vi "参考-分析生成报告文件.vi"(1 "最大缺陷面积":dbl, 2 "分析结果字符串":string[][](table), 3 "总缺陷面积":dbl, 4 "检测面  是否合格":string, 5 "请输入当前工件型号":string, 6 "时间":string) -> (0 "输出":string)   [LabVIEW 2018]
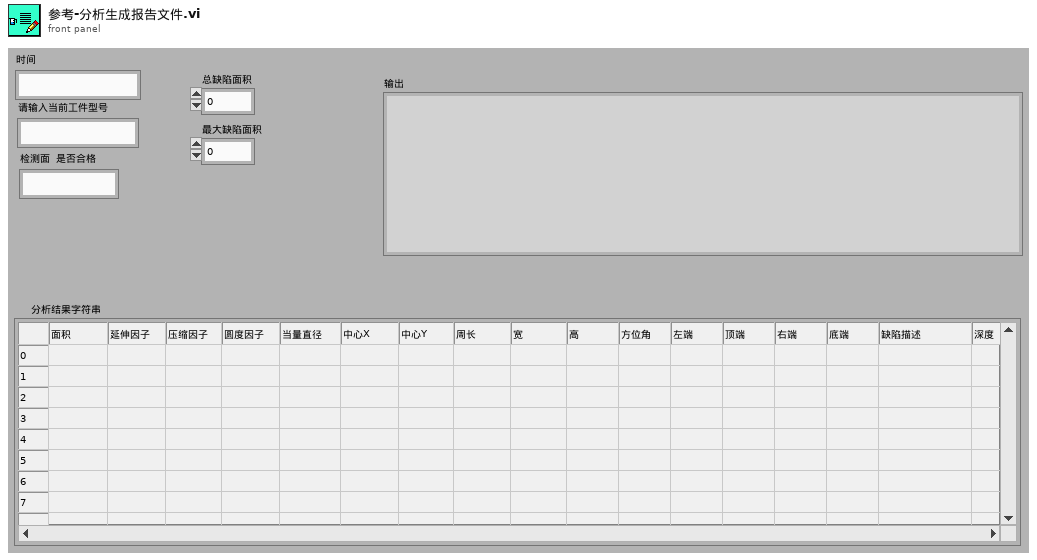
[diagram p1: front panel]
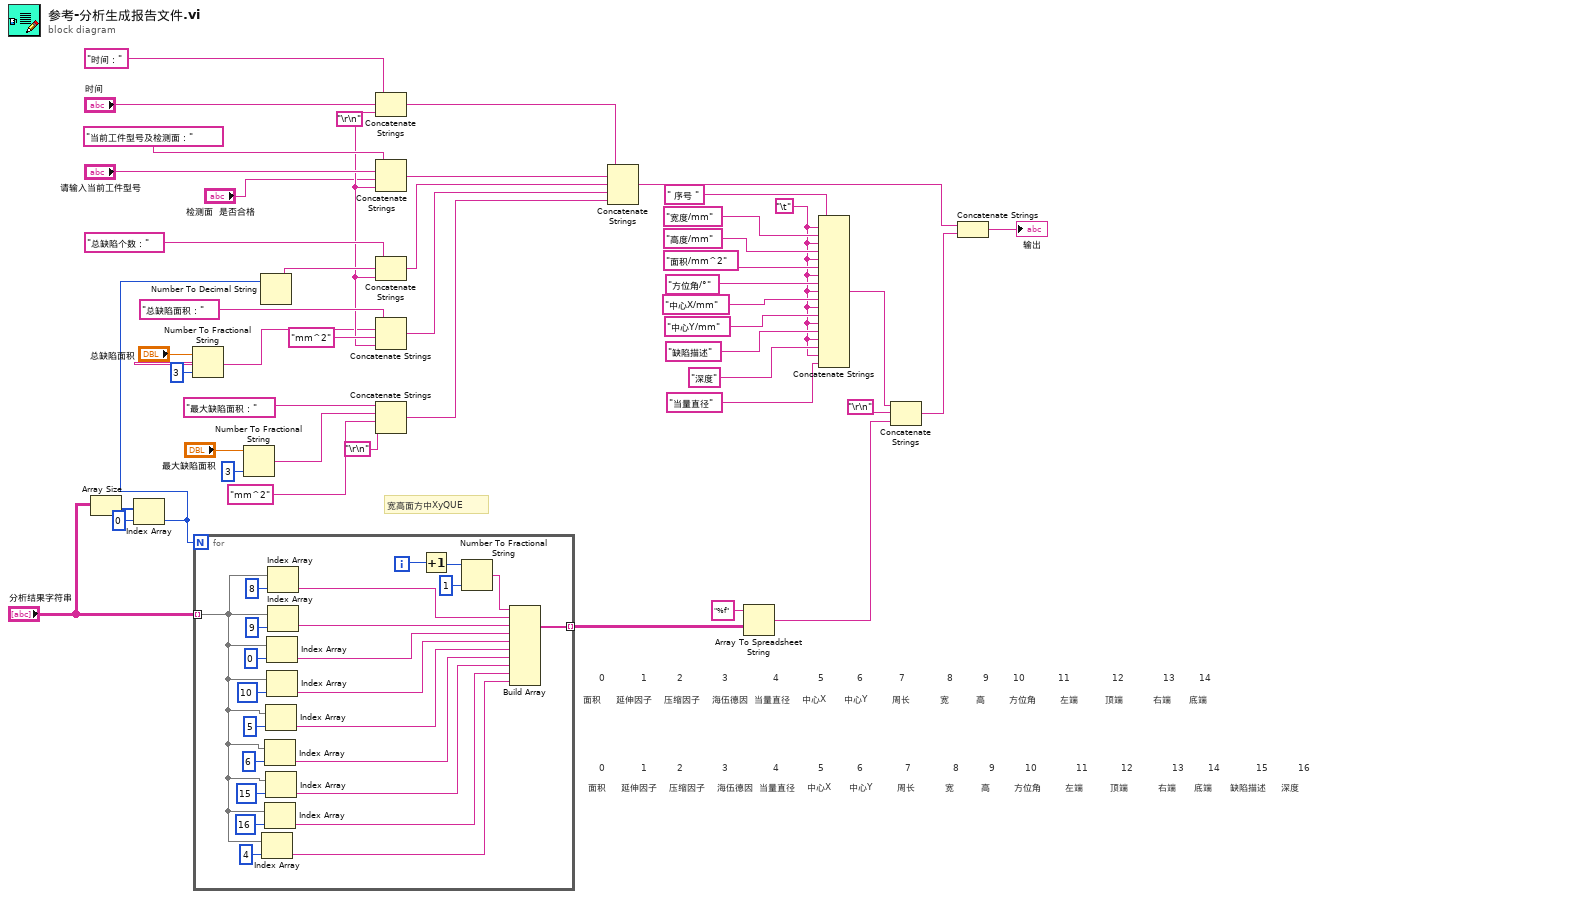
[diagram p0: block diagram]
diagram:
  w2 = "\t"
  w23 = "\r\n"
  # "面积     延伸因子    压缩因子    海伍德因  当量直径    中心X      中心Y        周长          宽         高        方位角        左端         顶端          右端      底端      缺陷描述     深度"
  # "0            1          2             3               4             5           6              7              8          9          10             11           12             13        14            15          16"
  # "面积     延伸因子    压缩因子    海伍德因  当量直径    中心X      中心Y        周长          宽         高        方位角        左端         顶端          右端      底端"
  # "0            1          2             3               4             5           6            7              8          9        10           11              12             13        14"
  # "宽高面方中XyQUE"
  n1 = Array Size(array="分析结果字符串") -> (size(s)=w6:i32[])
  n2 = Index Array(array=w6, index=0 ("索引")) -> (element=w4:i32)
  n3 = Number To Fractional String(number="总缺陷面积", precision (6)=i16 3) -> (F-format string=w20:string)  [unwired: 2 in]
  n4 = for {
    N: w4 -> [_]
    tunnel: [w71] -> w8 mode=indexing
    tunnel: "分析结果字符串" -> [w50] mode=indexing
    i -> [w70]
    n5 = Index Array(array=w50, index=4 ("索引")) -> (element=w49:string)
    n6 = Index Array(array=w50, index=6 ("索引")) -> (element=w55:string)
    n7 = Index Array(array=w50, index=16 ("索引")) -> (element=w48:string)
    n8 = Index Array(array=w50, index=5 ("索引")) -> (element=w56:string)
    n9 = Index Array(array=w50, index=15 ("索引")) -> (element=w53:string)
    n10 = Index Array(array=w50, index=0 ("索引")) -> (element=w61:string)
    n11 = Index Array(array=w50, index=10 ("索引")) -> (element=w59:string)
    n12 = Index Array(array=w50, index=8 ("索引")) -> (element=w64:string)
    n13 = Index Array(array=w50, index=9 ("索引")) -> (element=w63:string)
    n14 = Increment(x=w70) -> (x+1=w68:i32)
    n15 = Number To Fractional String(number=w68, precision (6)=1) -> (F-format string=w67:string)  [unwired: 2 in]
    n16 = Build Array(w67, w64, w63, w61, w59, w56, w55, w53, w48, w49) -> (w71:string[])
  }
  n17 = Number To Fractional String(number="最大缺陷面积", precision (6)=i16 3) -> (F-format string=w18:string)  [unwired: 2 in]
  n18 = Number To Decimal String(number=w4) -> (decimal integer string=w42:string)  [unwired: 1 in]
  n19 = Concatenate Strings("时间：", "时间", w23) -> (w41:string)
  n20 = Concatenate Strings("当前工件型号及检测面：", "请输入当前工件型号", "检测面  是否合格", w23) -> (w40:string)
  n21 = Concatenate Strings("总缺陷个数：", w42, w23) -> (w39:string)
  n22 = Concatenate Strings("总缺陷面积：", w20, "mm^2" ("string"), w23) -> (w26:string)
  n23 = Concatenate Strings("最大缺陷面积：", w18, "mm^2" ("string"), "\r\n") -> (w22:string)
  n24 = Concatenate Strings(w41, w40, w39, w26, w22) -> (w37:string)
  n25 = Array To Spreadsheet String(array=w8, 3:"%f") -> (spreadsheet string=w34:string)  [unwired: 1 in]
  n26 = Concatenate Strings(" 序号 ", w2, "宽度/mm", w2, "高度/mm", w2, "面积/mm^2", w2, "方位角/°", w2, "中心X/mm", w2, "中心Y/mm" ("string"), w2, "缺陷描述" ("字符串"), w2, "深度" ("字符串"), w2, "当量直径" ("字符串")) -> (w32:string)
  n27 = Concatenate Strings(w32, "\r\n", w34) -> (w36:string)
  n28 = Concatenate Strings(w37, w36) -> (→"输出":string)
